vi "Inverse Dynamics Demo.vi"() -> ()   [LabVIEW 2017, in "NI_Kinematics.lvlib"]
uses:
  <vilib>/robotics/Kinematics/NI_Kinematics.lvlib
  <vilib>/robotics/Kinematics/dyn/Inverse Dynamics (Trajectory).vi
  <vilib>/robotics/Kinematics/Generate Joint Trajectory (Array).vi
  <vilib>/robotics/Kinematics/Robot/NI_Robotics_Serial Robot Arm.lvclass
panel:
  out "Tau":dbl[][](array[numeric]) format="%#_6f"
  out "Time (ms)":u32
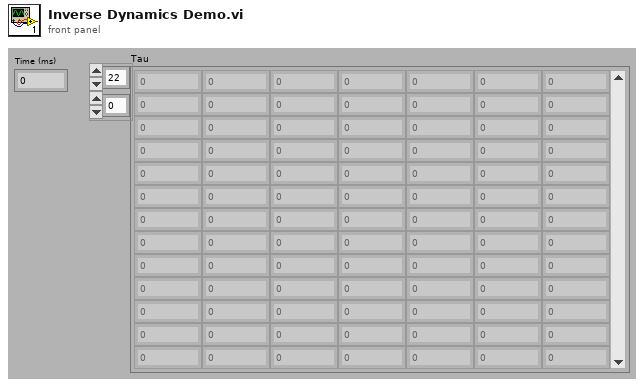
[diagram p1: front panel]
types:
  T1 = typedef "NI_Robotics_Serial Robot Arm.lvclass/Robot Pose.ctl" = cluster{"name":string, "description":string, "joint positions":dbl[]}
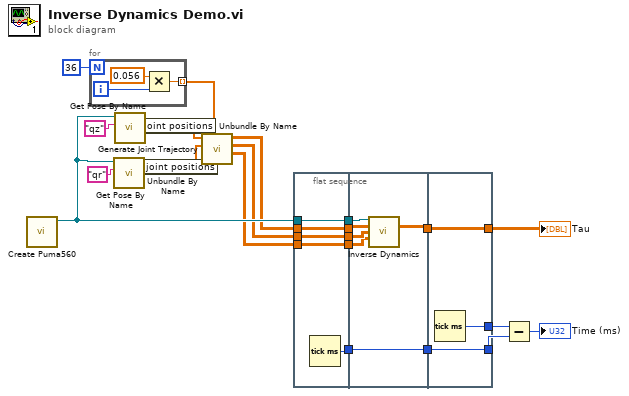
[diagram p0: block diagram]
diagram:
  n1 = call <vilib>:"Create Puma560.vi"() -> ("Puma560 Robot"=w13:refnum<class "NI_Robotics_Serial Robot Arm.lvclass">)  [unwired: 1 in, 10 out]
  n2 = for {
    N: 36 -> [_]
    tunnel: [w24] -> w1 mode=indexing
    i -> [w26]
    n3 = Multiply(x=0.056, y=w26) -> (x*y=w24:dbl)
  }
  n4 = call <vilib>:"Get Pose By Name.vi"("name"="qr" ("Name"), "serial arm in"=w13) -> ("serial arm pose"=w12:T1)  [unwired: 7 in, 2 out]
  n5 = call <vilib>:"Get Pose By Name.vi"("name"="qz" ("Name"), "serial arm in"=w13) -> ("serial arm pose"=w11:T1)  [unwired: 7 in, 2 out]
  n6 = Unbundle By Name(w11) -> ("joint positions"=w10:dbl[])
  n7 = Unbundle By Name(w12) -> ("joint positions"=w9:dbl[])
  n8 = call-poly <vilib>:"Generate Joint Trajectory.vi"("intermediate points"=w1, "end joint positions"=w9, "start joint positions"=w10) -> ("joint acceleration trajectory"=w6:dbl[][], "joint velocity trajectory"=w7:dbl[][], "joint position trajectory"=w8:dbl[][])  [unwired: 5 in, 1 out]
  n9 = flat-sequence {
    tunnel: w13 -> [w31]
    tunnel: [w31] -> w23
    tunnel: [w30] -> w22
    tunnel: w8 -> [w29]
    tunnel: w7 -> [w28]
    tunnel: w6 -> [w27]
    tunnel: [w29] -> w5
    tunnel: [w28] -> w4
    tunnel: [w27] -> w3
    tunnel: w23 -> [w36]
    tunnel: w22 -> [w37]
    tunnel: [w37] -> w21
    tunnel: [w32] -> w20
    tunnel: w5 -> [w35]
    tunnel: w4 -> [w34]
    tunnel: w3 -> [w33]
    tunnel: [w40] -> w18
    tunnel: w21 -> [w40]
    tunnel: [w39] -> w19
    tunnel: w20 -> [w38]
    tunnel: [w38] -> w16
    frame #0 {
      n10 = Tick Count (ms)() -> (millisecond timer value=w30:u32)
    }
    frame #1 {
      n11 = call-poly <vilib>:"Inverse Dynamics.vi"("serial arm in"=w36, "joint position trajectory"=w35, "joint velocity trajectory"=w34, "joint acceleration trajectory"=w33) -> ("required torque trajectory"=w32:dbl[][])  [unwired: 9 in, 2 out]
    }
    frame #2 {
      n12 = Tick Count (ms)() -> (millisecond timer value=w39:u32)
    }
  }
  n13 = Subtract(x=w19, y=w18) -> (x-y=→"Time (ms)":u32)
  "Tau" <- w16
